vi "Panela_R.vi"() -> ()   [LabVIEW 2017]
panel:
  in  "Panela_R":bool
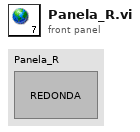
[diagram p1: front panel]
diagram:
